vi "Write XY position to file.vi"(4 "error in":errorcluster, 7 "refnum in":refnum<file>) -> (0 "error out":errorcluster, 3 "refnum out":refnum<file>)   [LabVIEW 2010]
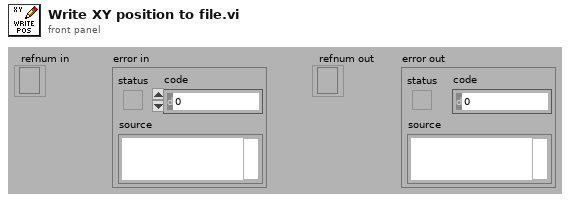
[diagram p1: front panel]
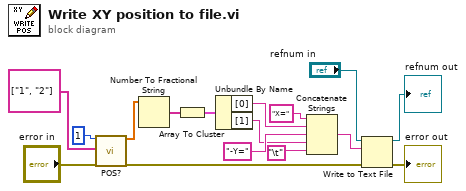
[diagram p0: block diagram]
diagram:
  n1 = call "POS?.vi"("System no."=1, "Axes to query"=string[] ["1", "2"], "error in"="error in") -> ("Position"=w4:dbl[], "error out"=w3:errorcluster)  [unwired: 15 in]
  n2 = Number To Fractional String(number=w4) -> (F-format string=w5:string[])  [unwired: 3 in]
  n3 = Array To Cluster(array=w5) -> (cluster=w10:cluster{"[0]":string, "[1]":string})
  n4 = Unbundle By Name(w10) -> ("[0]"=w8:string, "[1]"=w6:string)
  n5 = Concatenate Strings("X=" ("string"), w8, "-Y=" ("string"), w6, "\t") -> (w12:string)
  n6 = Write to Text File(file (use dialog)="refnum in", text=w12, error in=w3) -> (refnum out=→"refnum out":refnum<file>, error out=→"error out":errorcluster)  [unwired: 1 in, 1 out]
